vi "DAC Save Results.vi"(8 "error in":errorcluster, 9 "Log Details?":bool, 10 "tdms file":refnum<k34>, 11 "DAC HeatFlow AIV in":refnum<class "DAC HeatFlow AIV.lvclass">) -> (0 "error out":errorcluster)   [LabVIEW 2019, in "DAC.lvlib" / "DAC HeatFlow AIV.lvclass"]
uses:
  DAC HeatFlow AIV.lvclass
  C:/Users/krio/Documents/LV_Projects/test-stand/App/DAC/DAC.lvclass
  DAC.lvclass/DAC.ctl
  DAC HeatFlow AIV.lvclass/DAC HeatFlow AIV.ctl
  DAC.lvclass
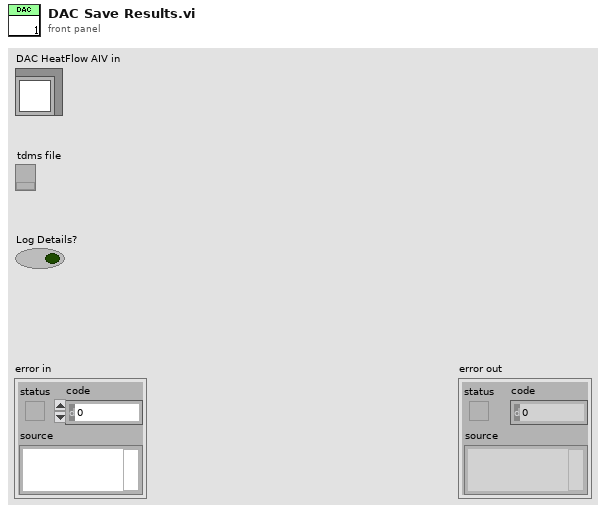
[diagram p1: front panel]
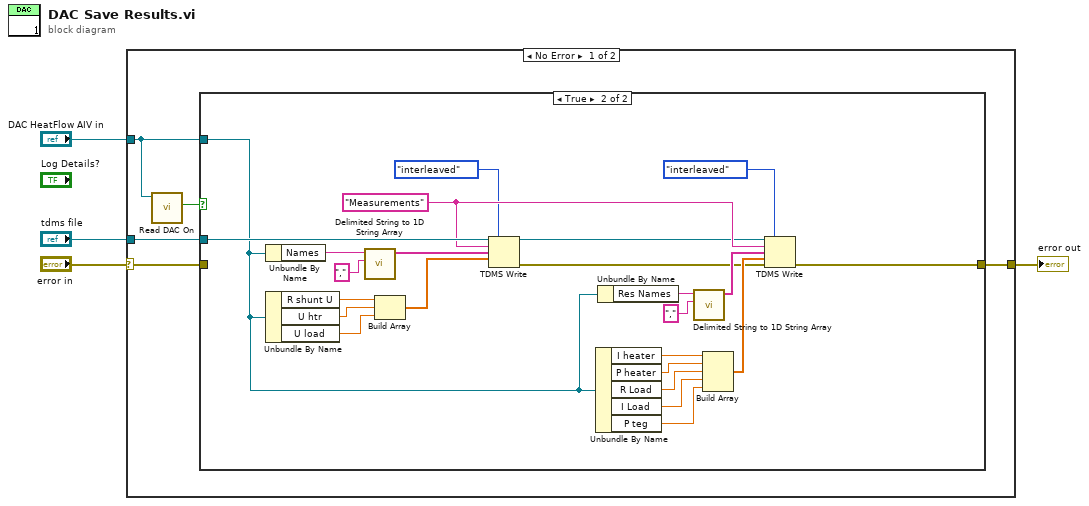
[diagram p0: block diagram]
diagram:
  n1 = case shown="No Error" "error in" {
    selector: "error in" -> [w6 w35]
    tunnel: "DAC HeatFlow AIV in" -> [w9 _]
    tunnel: "tdms file" -> [w7 _]
    tunnel: [w5 w35] -> w1
    frame No Error {
      n2 = call "Read DAC On.vi"("DAC in"=w9) -> ("DAC On"=w8:bool)  [unwired: 8 in, 2 out]
      n3 = case shown="True" w8 {
        tunnel: w9 -> [_ w14]
        tunnel: w7 -> [_ w34]
        tunnel: w6 -> [w10 _]
        tunnel: [w10 w22] -> w5
        frame False {
        }
        frame True {
          w33 = "Measurements" ("group name in (Untitled)")
          n4 = Unbundle By Name(w14) -> ("Names"=w20:string)
          n5 = Unbundle By Name(w14) -> ("R shunt U"=w19:dbl, "U htr"=w18:dbl, "U load"=w17:dbl)
          n6 = call <vilib>:"Delimited String to 1D String Array.vi"("delimiter"=",", "delimited string"=w20) -> ("string array"=w16:string[])  [unwired: 9 in]
          n7 = Build Array(w19, w18, w17) -> (w15:dbl[])
          n8 = TDMS Write(0:w34, 1:enum16{"decimated", "interleaved"}."interleaved" ("data layout (0:decimated)"), 5:w33, 7:w16, 9:w15) -> (4:w13:refnum<k34>, 15:w23:errorcluster)  [unwired: 1 in, 2 out]
          n9 = Unbundle By Name(w14) -> ("I heater"=w29:dbl, "P heater"=w28:dbl, "R Load"=w27:dbl, "I Load"=w26:dbl, "P teg"=w25:dbl)
          n10 = Unbundle By Name(w14) -> ("Res Names"=w31:string)
          n11 = call <vilib>:"Delimited String to 1D String Array.vi"("delimiter"=",", "delimited string"=w31) -> ("string array"=w30:string[])  [unwired: 9 in]
          n12 = Build Array(w29, w28, w27, w26, w25) -> (w24:dbl[])
          n13 = TDMS Write(0:w13, 1:enum16{"decimated", "interleaved"}."interleaved" ("data layout (0:decimated)"), 5:w33, 7:w30, 9:w24, 11:w23) -> (15:w22:errorcluster)  [unwired: 3 out]
        }
      }
    }
    frame Error {
    }
  }
  "error out" <- w1
